vi "Set Thread ID Pool.vi"(10 "Thread ID Pool":refnum<class "ID Pool.lvclass">, 11 "Transceiver Thread in":refnum<class "Transceiver Thread.lvclass">) -> (3 "Transceiver Thread out":refnum<class "Transceiver Thread.lvclass">)   [LabVIEW 2017, in "DSF Core.lvlib" / "Transceiver Thread.lvclass"]
uses:
  Transceiver Thread.lvclass
  Thread Pool/ID Pool.lvclass
  Transceiver Thread.lvclass/Transceiver Thread.ctl
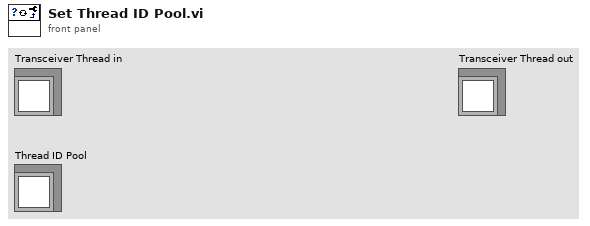
[diagram p1: front panel]
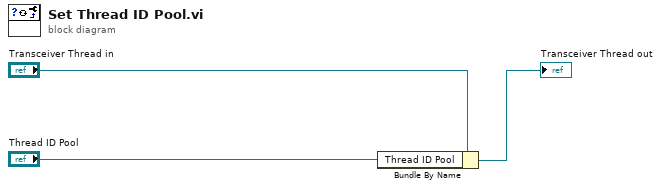
[diagram p0: block diagram]
diagram:
  n1 = Bundle By Name(cluster="Transceiver Thread in", "Thread ID Pool"="Thread ID Pool") -> (→"Transceiver Thread out":refnum<class "Transceiver Thread.lvclass">)
